vi "Add_TSL_Sweep_Speed.vi"(1 "TSL":refnum<k24>, 3 "error in (no error)":errorcluster) -> (8 "数组输出":string[](array[string]), 10 "error out":errorcluster)   [LabVIEW 2017]
doc: "' Add in selectable sweep speed to speed combbox\n ' this function can use only TSL-570"
uses:
  D:/test/PDLSTS/LV_PDL LvVer17.0/LV_PDL_x86/DLL/InstrumentDLL.dll
  DLL/InstrumentDLL.dll
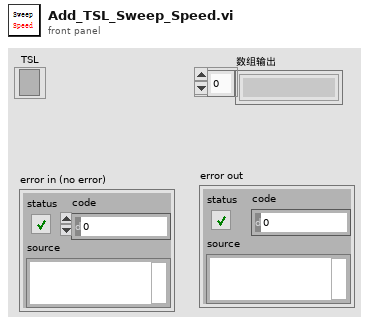
[diagram p1: front panel]
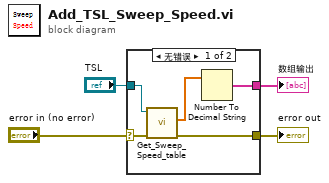
[diagram p0: block diagram]
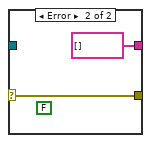
[diagram p2: hidden frame]
diagram:
  n1 = case shown="无错误" "error in (no error)" {
    selector: "error in (no error)" -> [w8 w11]
    tunnel: [w5 string[] []] -> w4
    tunnel: [w7 w11] -> w2
    tunnel: "TSL" -> [w9 _]
    frame No Error {
      n2 = call "Get_Sweep_Speed_table.vi"("error in (no error)"=w8, ".NET Reference in"=w9) -> ("error out"=w7:errorcluster, "Get_Sweep_Speed_table"=w6:dbl[])  [unwired: 7 in, 1 out]
      n3 = Number To Decimal String(number=w6) -> (decimal integer string=w5:string[])  [unwired: 1 in]
    }
    frame Error {
      (unwired) FALSE
    }
  }
  "数组输出" <- w4
  "error out" <- w2
